vi "plot_tree_control.vi"(8 "Point":T1, 9 "Plot Tree":refnum<vi>, 10 "Output File Loaded?":refnum<vi>) -> ()   [LabVIEW 2019]
uses:
  <vilib>/Utility/miscctls.llb/LVPositionTypeDef.ctl
panel:
  out "Blue":u32
  # "*******************************************************************\nBiogas Plant Control\n\nAuthor: Paul Zügel\nGCSC-Frankfurt am Main 2020\n\n*******************************************************************"
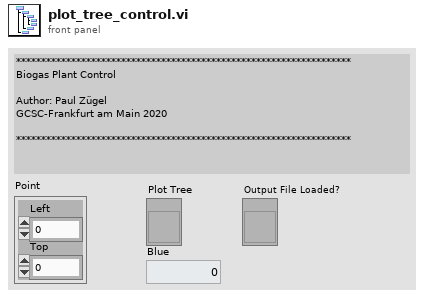
[diagram p1: front panel]
types:
  T1 = typedef "LVPositionTypeDef.ctl" = cluster{"Left":i32, "Top":i32}
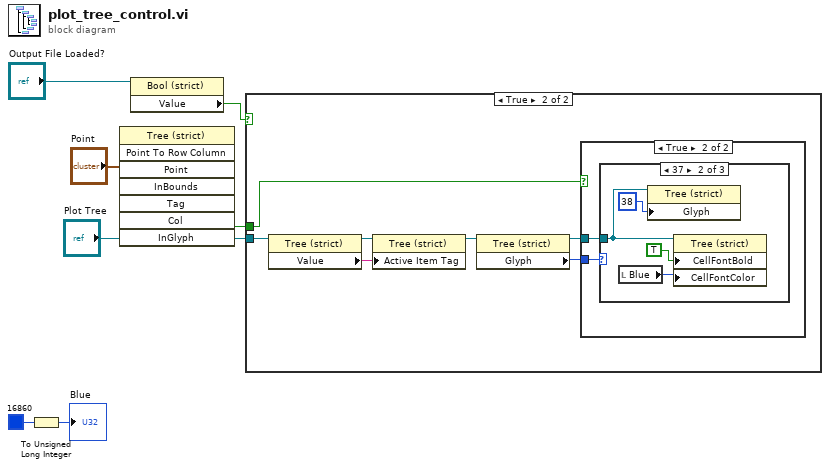
[diagram p0: block diagram]
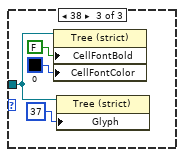
[diagram p5: hidden frame]
diagram:
  n1 = To Unsigned Long Integer(number=u32 16860) -> (unsigned 32bit integer=→"Blue":u32)
  n2 = invoke on="Invoke Node" class="Tree (strict)" method="Point To Row Column"(reference="Plot Tree", "Point"="Point") -> ("InGlyph"=w6:bool)  [unwired: 6 in, 7 out]
  n3 = property class="Bool (strict)"(reference="Output File Loaded?") -> ("Value"=w3:bool)  [unwired: 1 in, 2 out]
  n4 = case shown="True" w3 {
    tunnel: "Plot Tree" -> [_ w14]
    tunnel: w6 -> [_ w13]
    frame False {
    }
    frame True {
      n5 = property on="Property Node" class="Tree (strict)"(reference=w14) -> (reference out=w11:refnum<vi>, "Value"=w12:string)  [unwired: 1 in, 1 out]
      n6 = property on="Property Node" class="Tree (strict)"(reference=w11, "Active Item Tag"=w12) -> (reference out=w10:refnum<vi>)  [unwired: 1 in, 1 out]
      n7 = property on="Property Node" class="Tree (strict)"(reference=w10) -> (reference out=w9:refnum<vi>, "Glyph"=w8:i32)  [unwired: 1 in, 1 out]
      n8 = case shown="True" w13 {
        tunnel: w9 -> [_ w16]
        tunnel: w8 -> [_ w15]
        frame False {
        }
        frame True {
          n9 = case shown="37" w15 {
            tunnel: w16 -> [_ w19 w23]
            frame 15, Default {
            }
            frame 37 {
              n10 = local read "Blue"() -> (w17:u32)
              n11 = property on="Property Node" class="Tree (strict)"(reference=w19, "Glyph"=38 ("Active Item:Symbol Index")) -> ()  [unwired: 1 in, 2 out]
              n12 = property class="Tree (strict)"(reference=w19, "CellFontBold"=TRUE ("Active Cell:Cell Font:Bold"), "CellFontColor"=w17) -> ()  [unwired: 1 in, 2 out]
            }
            frame 38 {
              n13 = property class="Tree (strict)"(reference=w23, "CellFontBold"=FALSE ("Active Cell:Cell Font:Bold"), "CellFontColor"=u32 0 ("Active Cell:Cell Font:Color")) -> ()  [unwired: 1 in, 2 out]
              n14 = property on="Property Node" class="Tree (strict)"(reference=w23, "Glyph"=37 ("Active Item:Symbol Index")) -> ()  [unwired: 1 in, 2 out]
            }
          }
        }
      }
    }
  }
